vi "PH_ImageCalibrator.set Distance in Pixel.vi"(0 "i ref in":refnum<vi>, 5 "error in (no error)":errorcluster) -> (14 "i ref out":refnum<vi>, 19 "error out":errorcluster)   [LabVIEW 2014, in "PH_ImageCalibrator.lvlib"]
doc: "This VI pops up an auxiliary window to set a line. If set succesfully, die length of the line in calculated (in pixel) and set to the attributes. If this is not succesful or the cancel button pressed, the output Skip? is set to be true."
uses:
  PH_ImageCalibrator.lvlib
  PH_Basics/PH_Img_BaseClass/PH_Img_BaseClass.lvlib
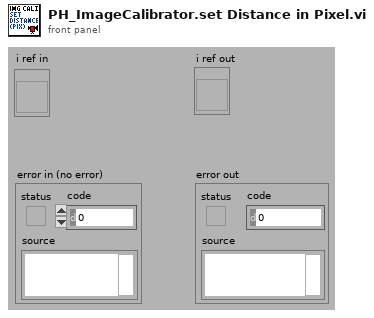
[diagram p1: front panel]
types:
  T1 = typedef "PH_ImageCalibrator.lvlib/PH_ImageCalibrator.i attribute.ctl" = cluster{"GUI Refs":cluster{"Available Cams":refnum<vi>, "OK":refnum<vi>, "Skip":refnum<vi>, "Repeat":refnum<vi>, "Cancel":refnum<vi>, "Length [mm]":refnum<vi>, "Energy [mJ]":refnum<vi>, "Dialog":refnum<vi>}, "Cam instances":string[], "Dark Pics":cluster{"#":i32, "BI taken":bool}, "Lin Cali":cluster{"Distance [Pixel]":dbl, "Distance [mm]":dbl, "Lin Cali Factor [mm/Pixel]":dbl}, "Energy Cali":cluster{"Pixelsum":dbl, "Energy [mJ]":dbl, "Energy Cali factor [mJ/Pixelsum]":dbl, "Underground subtracted?":bool, "#":i32}, "Images":cluster{"Background":T2, "Energy":T2}}
  T2 = typedef "IMAQ Image.ctl" = refnum<image>
  T3 = typedef "PH_Img_BaseClass.lvlib/PH_Img_BaseClass.i attribute.ctl" = cluster{"GUI Refs":T4, "Timeout Image [ms]":i32, "Default Periodic Period [ms]":i32, "Camera":cluster{"Instancename":string, "Notifier":refnum<notifier>}, "Palette":T5, "Cam Settings":cluster{"Cam ID":string, "Gain":dbl, "Brightness":dbl, "Shutter":dbl, "Cam Info Failure":bool, "Mode":i32}}
  T4 = typedef "PH_Img_BaseClass.lvlib/PH_Img_BaseClass.GUI Refs.ctl" = cluster{"Timeout":refnum<vi>, "Image":refnum<vi>, "Palette":refnum<vi>, "Timeout Set":refnum<vi>}
  T5 = typedef "PH_Img_BaseClass.lvlib/PH_Img_BaseClass.Palette.ctl" = i32
  T6 = cluster{"Global Rectangle":i32[], "Contours":cluster{"Contour Type":u32, "ROI Type":u32, "Points":i32[]}[]}
  T7 = cluster{"Contour Type":u32, "ROI Type":u32, "Points":i32[]}[]
  T8 = cluster{"Contour Type":u32, "ROI Type":u32, "Points":i32[]}
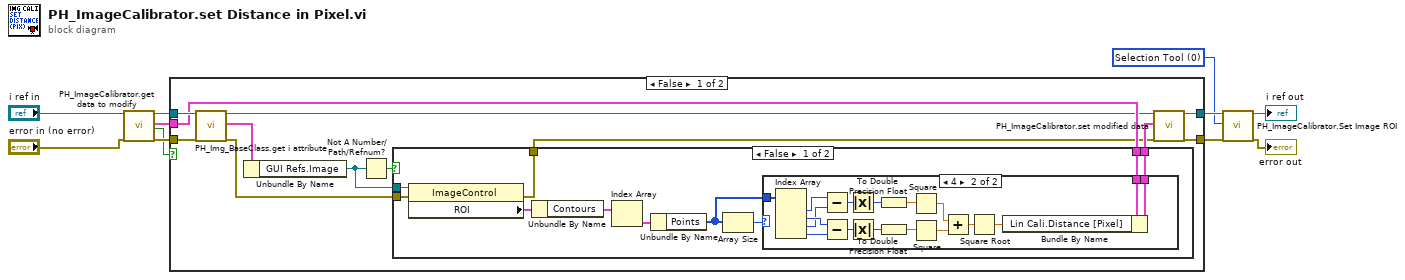
[diagram p0: block diagram]
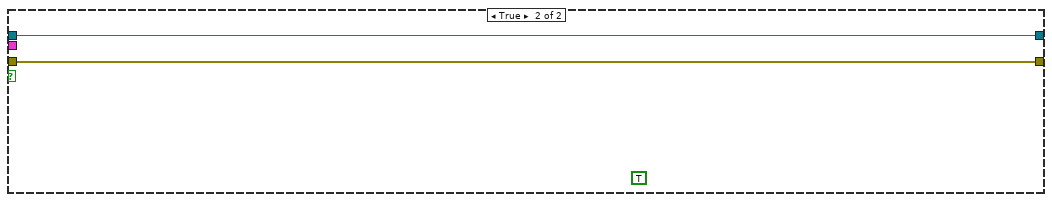
[diagram p4: hidden frame]
diagram:
  w1 = u32 0 items=["Zoom Tool"=8, "Selection Tool"=0, "Pan Tool"=9, "Point Tool"=1, "Line Tool"=2, "Rectangle Tool"=3, "Rotated Rectangle Tool"=12, "Polyline Tool"=10, "Polygon Tool"=5, "Freehand Tool"=11, "Closed Freehand Tool"=6, "Ellipse Tool"=4, "Annulus Tool"=7] ("ROI Tool")
  n1 = call "PH_ImageCalibrator.get data to modify.vi"("i ref in"="i ref in", "error in (no error)"="error in (no error)") -> ("i ref out"=w9:refnum<vi>, "i attribute"=w11:T1, "timed out"=w6:bool, "error out"=w10:errorcluster)  [unwired: 14 in]
  n2 = case shown="False" w6 {
    tunnel: w9 -> [w23 w55]
    tunnel: w10 -> [w14 w54]
    tunnel: w11 -> [w19 _]
    tunnel: [w21 w54] -> w4
    tunnel: [w20 w55] -> w5
    frame False {
      n3 = call "PH_Img_BaseClass.get i attribute.vi"("i ref in"=w23, "error in (no error)"=w14) -> ("i ref out"=w15:refnum<vi>, "i attribute"=w12:T3, "error out"=w13:errorcluster)  [unwired: 15 in]
      n4 = Unbundle By Name(w12) -> ("GUI Refs.Image"=w17:refnum<vi>)
      n5 = Not A Number/Path/Refnum?(number/path/refnum=w17) -> (NaN/Path/Refnum?=w16:bool)
      n6 = case shown="False" w16 {
        tunnel: [w33 w52] -> w22
        tunnel: w19 -> [w32 w52]
        tunnel: w17 -> [w31 _]
        tunnel: [w27 w53] -> w18
        tunnel: w13 -> [w26 w53]
        frame False {
          n7 = property class="ImageControl"(reference=w31, error in=w26) -> (error out=w27:errorcluster, "ROI"=w30:T6)  [unwired: 1 out]
          n8 = Unbundle By Name(w30) -> ("Contours"=w29:T7)
          n9 = Index Array(array=w29) -> (element=w28:T8)  [unwired: 1 in]
          n10 = Unbundle By Name(w28) -> ("Points"=w25:i32[])
          n11 = Array Size(array=w25) -> (size(s)=w24:i32)
          n12 = case shown="4" w24 {
            tunnel: [w34 w51] -> w33
            tunnel: w32 -> [w34 w50]
            tunnel: w25 -> [_ w37]
            frame Default {
            }
            frame 4 {
              n13 = Index Array(array=w37) -> (element #1=w46:i32, element #2=w48:i32, element #3=w47:i32, element #4=w49:i32)  [unwired: 4 in]
              n14 = Subtract(x=w46, y=w47) -> (x-y=w40:i32)
              n15 = Subtract(x=w48, y=w49) -> (x-y=w43:i32)
              n16 = Absolute Value(x=w40) -> (abs(x)=w41:i32)
              n17 = Absolute Value(x=w43) -> (abs(x)=w44:i32)
              n18 = To Double Precision Float(number=w41) -> (double precision float=w35:dbl)
              n19 = To Double Precision Float(number=w44) -> (double precision float=w36:dbl)
              n20 = Square(x=w35) -> (x^2=w42:dbl)
              n21 = Square(x=w36) -> (x^2=w45:dbl)
              n22 = Add(x=w42, y=w45) -> (x+y=w39:dbl)
              n23 = Square Root(x=w39) -> (sqrt(x)=w38:dbl)
              n24 = Bundle By Name(cluster=w50, "Lin Cali.Distance [Pixel]"=w38) -> (w51:T1)
            }
          }
        }
        frame True {
        }
      }
      n25 = call "PH_ImageCalibrator.set modified data.vi"("i ref in"=w15, "i attribute"=w22, "error in (no error)"=w18) -> ("i ref out"=w20:refnum<vi>, "error out"=w21:errorcluster)  [unwired: 15 in]
    }
    frame True {
      (unwired) TRUE ("Cancelled")
    }
  }
  n26 = call "PH_ImageCalibrator.Set Image ROI.vi"("i ref in"=w5, "ROI Tool"=w1, "error in"=w4) -> ("i ref out"=→"i ref out":refnum<vi>, "error out"=→"error out":errorcluster)  [unwired: 15 in]
